vi "Enqueue_Data.vi"(8 "error in (no error)":errorcluster, 11 "Ref in":T1 {"TS Parameter"."FCA" format="%01d"; "TS Parameter"."Target" min=1 max=100000; "TS Parameter"."PokaYoke" min=0 max=1}) -> (0 "error out":errorcluster, 3 "Ref out":T1 {"TS Parameter"."FCA" format="%01d"; "TS Parameter"."Target" min=1 max=100000; "TS Parameter"."PokaYoke" min=0 max=1})   [LabVIEW 2020]
uses:
  Controls/TD SQL.ctl
  <vilib>/addons/database/Connection.llb/Conn ObjectReference.ctl
  Controls/WIP_State.ctl
  Controls/TS_Parameter.ctl
  <vilib>/addons/database/NI_Database_API.lvlib
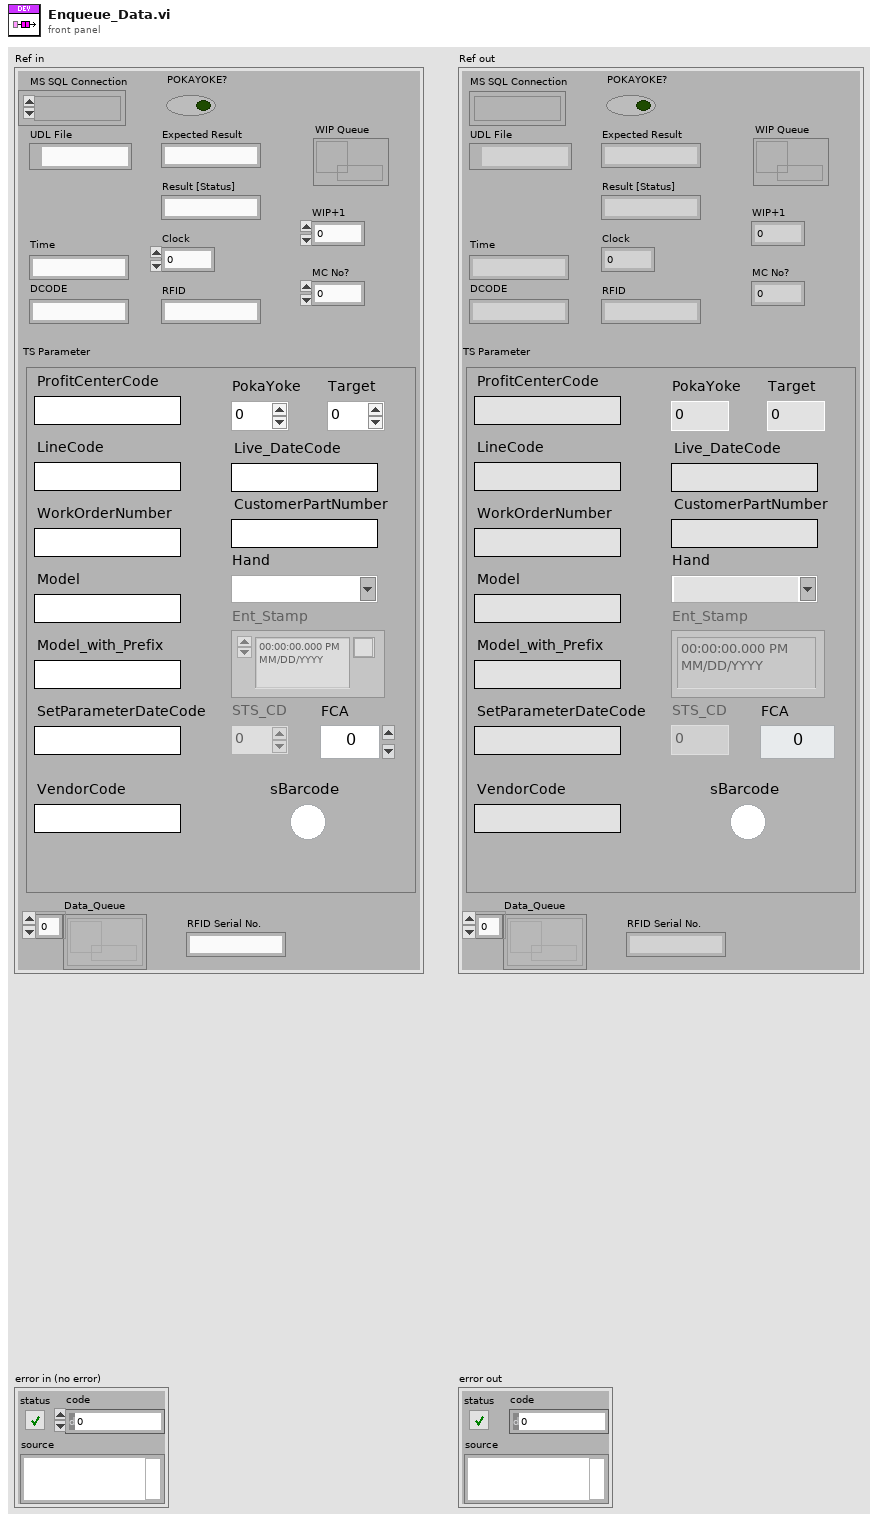
[diagram p1: front panel]
types:
  T1 = typedef "TD SQL.ctl" = cluster{"MS SQL Connection":T2, "UDL File":path, "Time":string, "DCODE":string, "WIP+1":i64, "MC No?":i32, "POKAYOKE?":bool, "Expected Result":string, "Result [Status]":string, "Clock":dbl, "RFID":string, "WIP Queue":refnum<queue>, "TS Parameter":T3, "Data_Queue":refnum<queue>[], "RFID Serial No.":string}
  T2 = typedef "NI_Database_API.lvlib/Conn ObjectReference.ctl" = refnum<k1>
  T3 = typedef "TS_Parameter.ctl" = cluster{"ProfitCenterCode":string, "LineCode":string, "WorkOrderNumber":string, "Model":string, "Model_with_Prefix":string, "VendorCode":string, "SetParameterDateCode":string, "PokaYoke":i32, "Target":i32, "Live_DateCode":string, "CustomerPartNumber":string, "Hand":string, "sBarcode":bool, "FCA":i32, "Ent_Stamp":timestamp, "STS_CD":dbl}
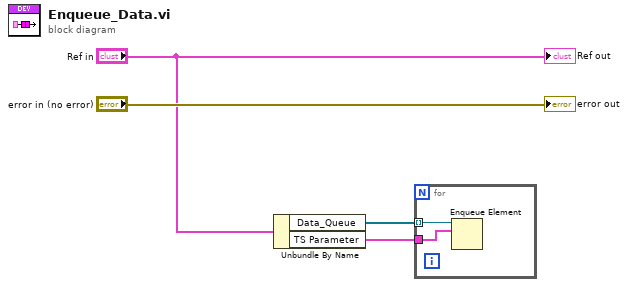
[diagram p0: block diagram]
diagram:
  n1 = Unbundle By Name("Ref in") -> ("Data_Queue"=w2:refnum<queue>[], "TS Parameter"=w1:T3)
  n2 = for {
    tunnel: w2 -> [w6] mode=indexing
    tunnel: w1 -> [w5]
    n3 = Enqueue Element(queue=w6, element=w5) -> ()  [unwired: 2 in, 3 out]
  }
  "error out" <- "error in (no error)"
  "Ref out" <- "Ref in"
